vi "Tree Empty.vi"(0 "Tree Reference In":refnum<vi>, 5 "error in (no error)":errorcluster, 8 "Return Elements":bool) -> (14 "Tree Reference Out":refnum<vi>, 16 "Deleted Tree Items":string[](array[string]), 19 "error out":errorcluster)   [LabVIEW 2014]
doc: "Deletes all elements from<B>Tree Reference In</B>. Passes deleted elements from the tree out in a 1-D array. The array is ordered top to bottom item as they were in the tree."
panel:
  # "VI INPUTS"
  # "VI OUTPUTS"
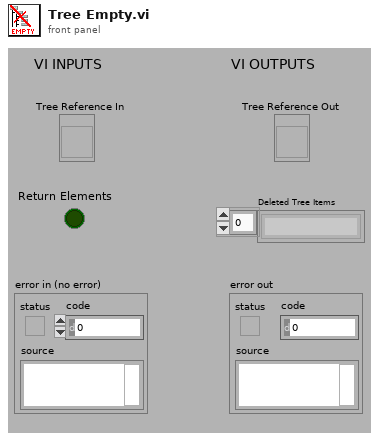
[diagram p1: front panel]
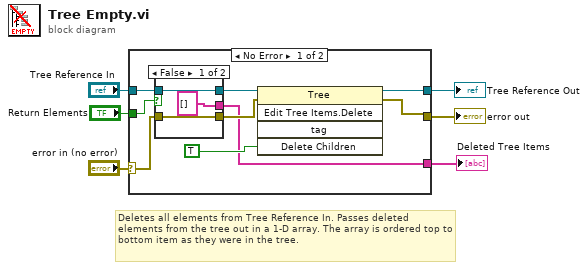
[diagram p0: block diagram]
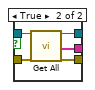
[diagram p2: hidden frame]
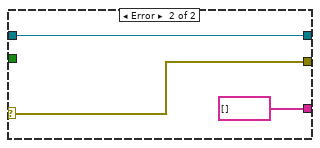
[diagram p3: hidden frame]
diagram:
  # "Deletes all elements from Tree Reference In. Passes deleted elements from the tree out in a 1-D array. The array is ordered top to bottom item as they were in the tree."
  n1 = case shown="No Error" "error in (no error)" {
    selector: "error in (no error)" -> [w14 w25]
    tunnel: "Tree Reference In" -> [w15 w26]
    tunnel: [w12 w26] -> w5
    tunnel: [w9 w25] -> w4
    tunnel: [w8 string[] []] -> w2
    tunnel: "Return Elements" -> [w7 _]
    frame No Error {
      n2 = case shown="False" w7 {
        tunnel: w15 -> [w17 w23]
        tunnel: w14 -> [w18 w22]
        tunnel: [string[] [] ("Output Tree Items") w21] -> w8
        tunnel: [w17 w20] -> w13
        tunnel: [w18 w19] -> w11
        frame False {
        }
        frame True {
          n3 = call "Get All.vi"("Tree Reference In"=w23, "error in (no error)"=w22) -> ("Tree Reference Out"=w20:refnum<vi>, "Output Tree Items"=w21:string[], "error out"=w19:errorcluster)  [unwired: 14 in, 1 out]
        }
      }
      n4 = invoke class="Tree" method="Edit Tree Items.Delete"(reference=w13, error in=w11, "Delete Children"=TRUE) -> (reference out=w12:refnum<vi>, error out=w9:errorcluster)  [unwired: 2 in, 3 out]
    }
    frame Error {
    }
  }
  "Tree Reference Out" <- w5
  "error out" <- w4
  "Deleted Tree Items" <- w2
